vi "Data Server Decode Command.vi"(5 "Corrector names":string[](array[string])=["ACH01B", "ACH02", "ACH03B", "ACH04", "ACH05A", "ACH06", "ACH07A", "ACH07B", "ACH08"], 7 "BPM names":string[](array[string])=["ACH01B", "ACH02", "ACH03B", "ACH04", "ACH05A", "ACH06", "ACH07A", "ACH07B", "ACH08"], 8 "error in (no error)":errorcluster, 11 "Input string":string) -> (0 "error out":errorcluster, 1 "BPM and PS index":T2, 2 "Number of samples":u32, 3 "Filename":string, 4 "Command ID":T1=enum."FA_Start")   [LabVIEW 2011, in "Data Server VIs.lvlib"]
uses:
  Data Server VIs.lvlib
  Types Definitions/Type BPM and PS select cluster.ctl
  Types Definitions/Type Data Server Command ID.ctl
  Type Definitions.lvlib
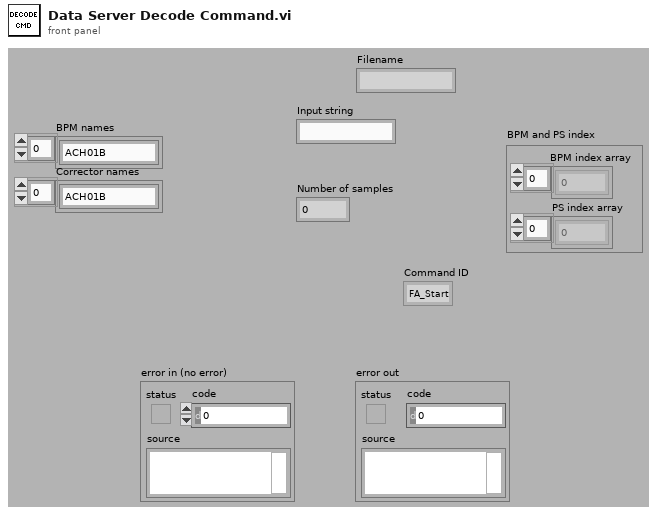
[diagram p1: front panel]
types:
  T1 = typedef "Type Definitions.lvlib/Type Data Server Command ID.ctl" = enum16{"None", "FA_Start", "FA_Stop", "Update_Controller"}
  T2 = typedef "Type Definitions.lvlib/Type BPM and PS select cluster.ctl" = cluster{"BPM index array":u32[], "PS index array ":u32[]}
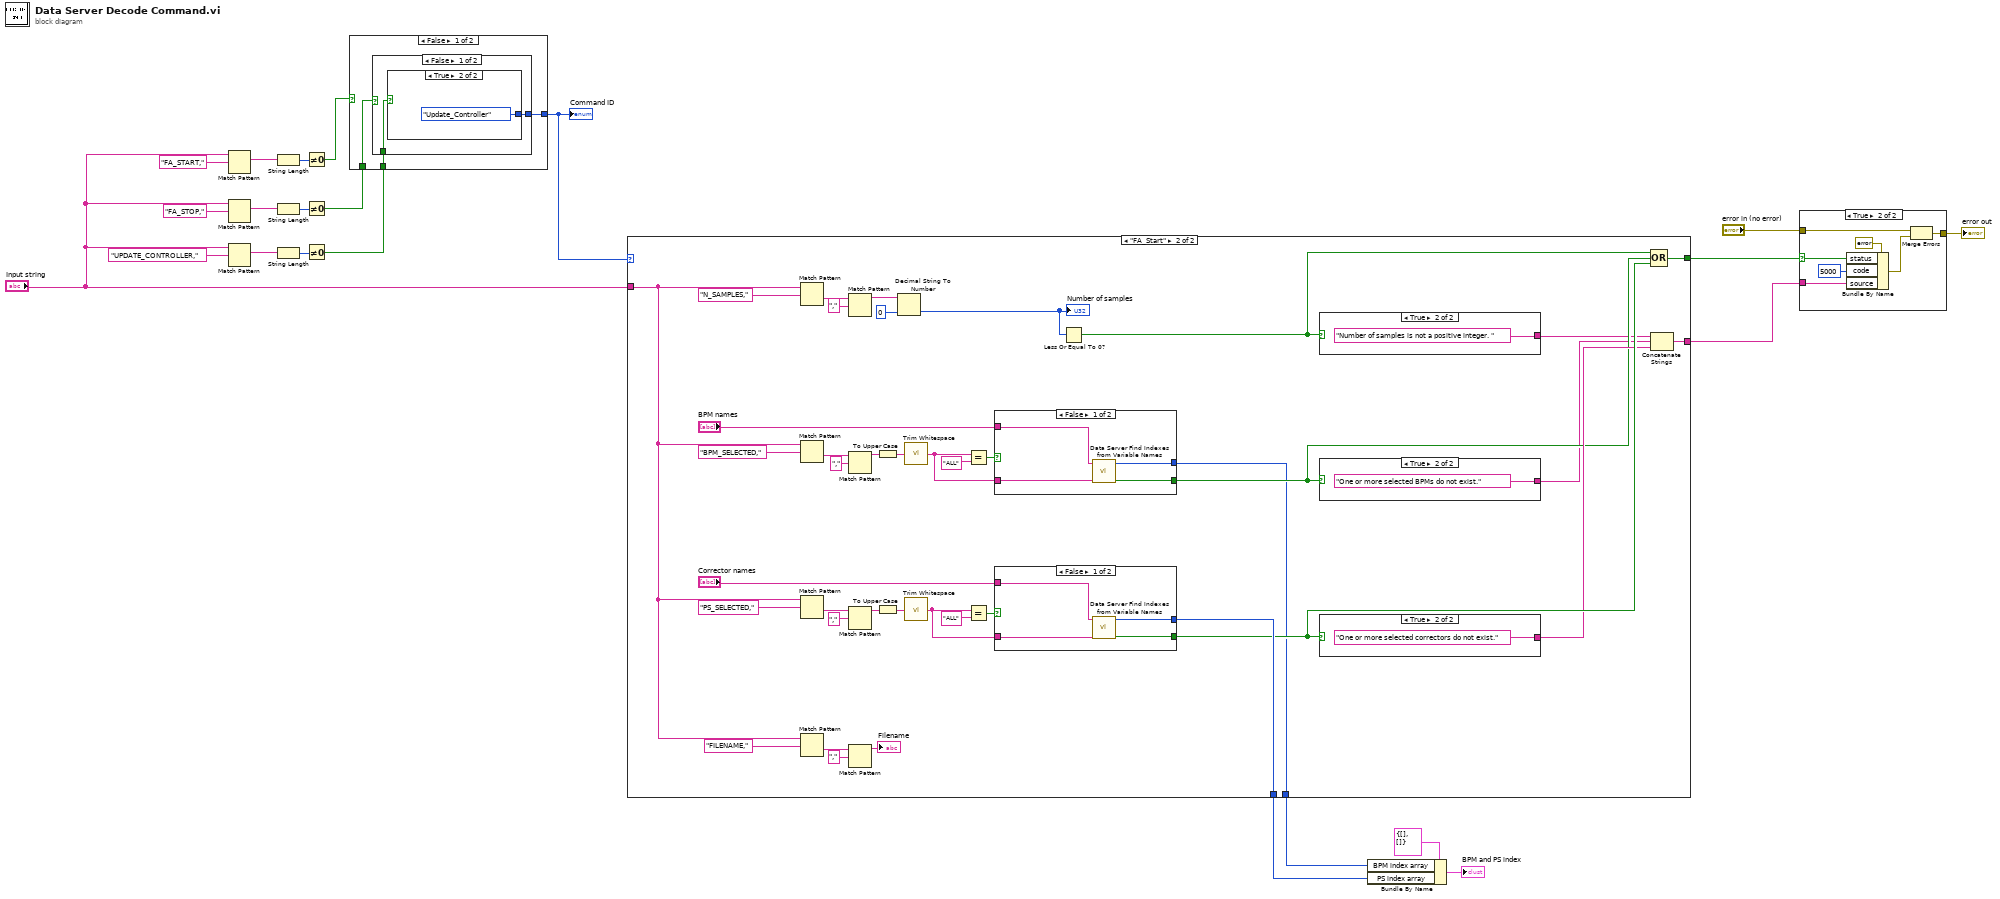
[diagram p0: block diagram]
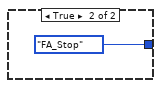
[diagram p3: hidden frame]
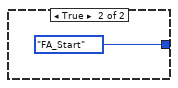
[diagram p4: hidden frame]
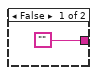
[diagram p6: hidden frame]
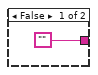
[diagram p7: hidden frame]
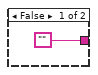
[diagram p8: hidden frame]
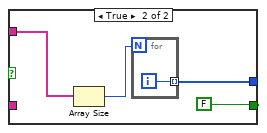
[diagram p9: hidden frame]
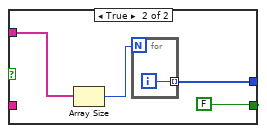
[diagram p10: hidden frame]
diagram:
  n1 = Match Pattern(string="Input string", regular expression="FA_START,") -> (match substring=w9:string)  [unwired: 1 in, 3 out]
  n2 = Match Pattern(string="Input string", regular expression="FA_STOP,") -> (match substring=w15:string)  [unwired: 1 in, 3 out]
  n3 = Match Pattern(string="Input string", regular expression="UPDATE_CONTROLLER,") -> (match substring=w5:string)  [unwired: 1 in, 3 out]
  n4 = String Length(string=w9) -> (length=w10:i32)
  n5 = String Length(string=w15) -> (length=w14:i32)
  n6 = String Length(string=w5) -> (length=w6:i32)
  n7 = Not Equal To 0?(x=w10) -> (x != 0?=w8:bool)
  n8 = Not Equal To 0?(x=w14) -> (x != 0?=w7:bool)
  n9 = Not Equal To 0?(x=w6) -> (x != 0?=w2:bool)
  n10 = case shown="False" w8 {
    tunnel: w7 -> [w25 _]
    tunnel: [w24 Type_Data_Server_Command_ID."FA_Start"] -> w1
    tunnel: w2 -> [w23 _]
    frame False {
      n11 = case shown="False" w25 {
        tunnel: [w27 Type_Data_Server_Command_ID."FA_Stop"] -> w24
        tunnel: w23 -> [w26 _]
        frame False {
          n12 = case shown="True" w26 {
            tunnel: [_ Type_Data_Server_Command_ID."Update_Controller"] -> w27
            frame False {
            }
            frame True {
            }
          }
        }
        frame True {
        }
      }
    }
    frame True {
    }
  }
  "Command ID" <- w1
  n13 = case shown="\"FA_Start\"" w1 {
    tunnel: [_ w49] -> w20
    tunnel: [_ w46] -> w12
    tunnel: [_ w39] -> w17
    tunnel: [_ w38] -> w13
    tunnel: "Input string" -> [_ w32]
    frame "None", Default {
    }
    frame "FA_Start" {
      n14 = Match Pattern(string=w32, regular expression="N_SAMPLES,") -> (after substring=w68:string)  [unwired: 1 in, 3 out]
      n15 = Match Pattern(string=w32, regular expression="BPM_SELECTED,") -> (after substring=w62:string)  [unwired: 1 in, 3 out]
      n16 = Match Pattern(string=w32, regular expression="PS_SELECTED,") -> (after substring=w52:string)  [unwired: 1 in, 3 out]
      n17 = Match Pattern(string=w32, regular expression="FILENAME,") -> (after substring=w34:string)  [unwired: 1 in, 3 out]
      n18 = Match Pattern(string=w68, regular expression=",") -> (before substring=w66:string)  [unwired: 1 in, 3 out]
      n19 = Match Pattern(string=w62, regular expression=",") -> (before substring=w50:string)  [unwired: 1 in, 3 out]
      n20 = Match Pattern(string=w52, regular expression=",") -> (before substring=w54:string)  [unwired: 1 in, 3 out]
      n21 = Match Pattern(string=w34, regular expression=",") -> (before substring=→"Filename":string)  [unwired: 1 in, 3 out]
      n22 = To Upper Case(1:w50) -> (0:w59:string)
      n23 = To Upper Case(1:w54) -> (0:w56:string)
      n24 = Decimal String To Number(string=w66, default (0L)=u32 0 ("y")) -> (number=w64:u32)  [unwired: 1 in, 1 out]
      "Number of samples" <- w64
      n25 = call <vilib>:"Trim Whitespace.vi"("string"=w59) -> ("trimmed string"=w57:string)  [unwired: 1 in]
      n26 = call <vilib>:"Trim Whitespace.vi"("string"=w56) -> ("trimmed string"=w48:string)  [unwired: 1 in]
      n27 = Equal?(x=w57, y="ALL") -> (x = y?=w58:bool)
      n28 = Equal?(x=w48, y="ALL") -> (x = y?=w47:bool)
      n29 = case shown="False" w58 {
        tunnel: w57 -> [w88 _]
        tunnel: [w86 w89] -> w38
        tunnel: [w85 FALSE ("Index Fault")] -> w43
        tunnel: "BPM names" -> [w87 w90]
        frame False {
          n30 = call "Data Server Find Indexes from Variable Names.vi"("Comand string"=w88, "Variable names"=w87) -> ("Command error"=w85:bool, "Index array"=w86:i32[])  [unwired: 8 in]
        }
        frame True {
          n31 = Array Size(array=w90) -> (size(s)=w91:i32)
          n32 = for {
            N: w91 -> [_]
            tunnel: [w93] -> w89 mode=indexing
            i -> [w93]
          }
        }
      }
      n33 = case shown="False" w47 {
        tunnel: w48 -> [w77 _]
        tunnel: [w78 w80] -> w46
        tunnel: [w76 FALSE ("Index Fault")] -> w45
        tunnel: "Corrector names" -> [w79 w81]
        frame False {
          n34 = call "Data Server Find Indexes from Variable Names.vi"("Comand string"=w77, "Variable names"=w79) -> ("Command error"=w76:bool, "Index array"=w78:i32[])  [unwired: 8 in]
        }
        frame True {
          n35 = Array Size(array=w81) -> (size(s)=w82:i32)
          n36 = for {
            N: w82 -> [_]
            tunnel: [w84] -> w80 mode=indexing
            i -> [w84]
          }
        }
      }
      n37 = Less Or Equal To 0?(x=w64) -> (x <= 0?=w42:bool)
      n38 = case shown="True" w42 {
        tunnel: ["" "Number of samples is not a positive integer. "] -> w41
        frame False {
        }
        frame True {
        }
      }
      n39 = case shown="True" w43 {
        tunnel: ["" "One or more selected BPMs do not exist."] -> w40
        frame False {
        }
        frame True {
        }
      }
      n40 = case shown="True" w45 {
        tunnel: ["" "One or more selected correctors do not exist."] -> w44
        frame False {
        }
        frame True {
        }
      }
      n41 = Compound Arithmetic op=OR(w42, w43, w45) -> (w49:bool)
      n42 = Concatenate Strings(w41, w40, w44) -> (w39:string)
    }
  }
  n43 = Bundle By Name(cluster=T2 {"BPM index array"=[], "PS index array "=[]} ("Cluster"), "BPM index array"=w13, "PS index array"=w12) -> (→"BPM and PS index":T2)
  n44 = case shown="True" w20 {
    selector: w20 -> [_ w95]
    tunnel: "error in (no error)" -> [w94 w99]
    tunnel: [w94 w97] -> w21
    tunnel: w17 -> [_ w96]
    frame False {
    }
    frame True {
      n45 = Bundle By Name(cluster=errorcluster {"status"=TRUE, "code"=0, "source"=""} ("error out"), "status"=w95, "code"=5000, "source"=w96) -> (w98:errorcluster)
      n46 = Merge Errors(w99, w98) -> (w97:errorcluster)
    }
  }
  "error out" <- w21
